vi "Check Feature Toggle.vi"(8 "error in (no error)":errorcluster, 11 "feature name":string) -> (0 "error out":errorcluster, 3 "feature enabled":bool)   [LabVIEW 2020, in "Engine Simulation Toolkit System Explorer.lvlib"]
uses:
  Engine Simulation Toolkit System Explorer.lvlib
  NationalInstruments.VeriStand.SystemDefinitionAPI
  <vilib>/Utility/config.llb/Read Key (Boolean).vi
  <vilib>/Utility/config.llb/NI_LVConfig.lvlib
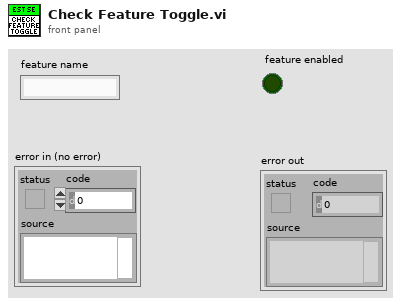
[diagram p1: front panel]
types:
  T1 = typedef "NI_LVConfig.lvlib/Config Data RefNum.ctl" = refnum<k1>
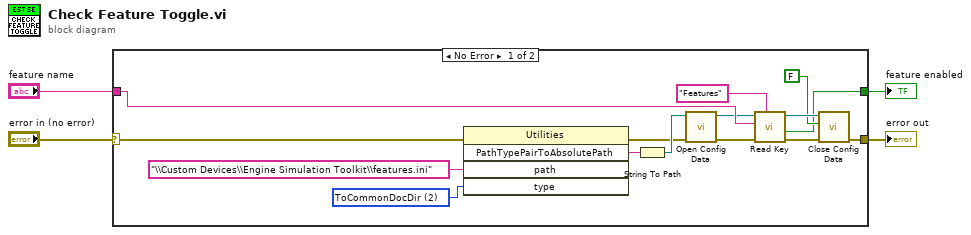
[diagram p0: block diagram]
diagram:
  n1 = case shown="No Error" "error in (no error)" {
    selector: "error in (no error)" -> [w7 w20]
    tunnel: [w16 w20] -> w4
    tunnel: "feature name" -> [w13 _]
    tunnel: [w14 _] -> w1
    frame No Error {
      w11 = 2 items=["Absolute", "ToBase", "ToCommonDocDir", "ToApplicationDataDir"] ("type")
      n2 = invoke class="Utilities" method="PathTypePairToAbsolutePath"(error in=w7, "path"="\\Custom Devices\\Engine Simulation Toolkit\\features.ini", "type"=w11) -> (error out=w8:errorcluster, "PathTypePairToAbsolutePath"=w10:string)  [unwired: 2 in, 3 out]
      n3 = String To Path(string=w10) -> (path=w9:path)
      n4 = call <vilib>:"Open Config Data.vi"("error in (no error)"=w8, "configuration file path"=w9) -> ("error out"=w17:errorcluster, "refnum"=w6:T1)  [unwired: 7 in, 1 out]
      n5 = call-poly <vilib>:"Read Key.vi"("section"="Features", "error in (no error)"=w17, "key"=w13, "refnum"=w6) -> ("error out"=w18:errorcluster, "value"=w14:bool, "refnum out"=w19:T1)  [unwired: 4 in, 1 out]
      n6 = call <vilib>:"Close Config Data.vi"("error in (no error)"=w18, "write file if changed (T)"=FALSE, "refnum"=w19) -> ("error out"=w16:errorcluster)  [unwired: 7 in, 1 out]
    }
    frame Error {
    }
  }
  "feature enabled" <- w1
  "error out" <- w4
